vi "Qrcode Scanner Array Split.vi"() -> ()   [LabVIEW 2019]
uses:
  <vilib>/userDefined/High Color/IMAQdx.ctl
  <vilib>/vision/driver/NI_Vision_Acquisition_Software.lvlib
  <vilib>/vision/NI_Vision_Development_Module.lvlib
panel:
  out "Array":string[](array[string])
  in  "Session In":T1
  out "Found?":bool
  out "Image":T2(plugin-control)
  out "Data":string
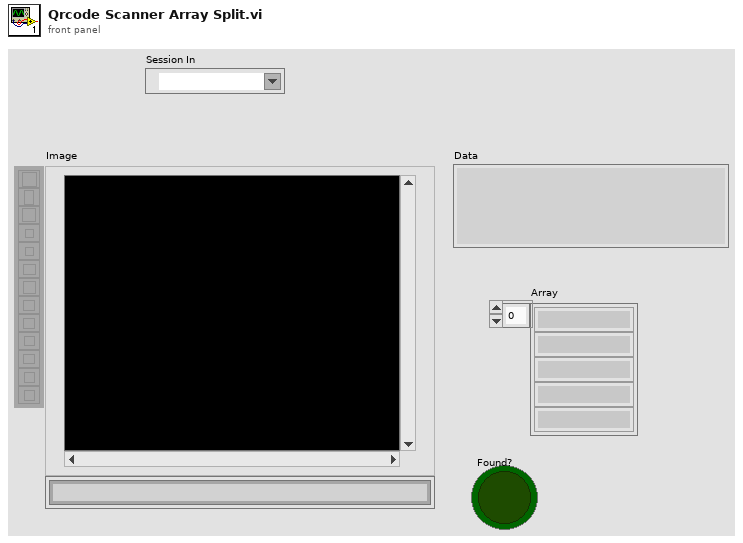
[diagram p1: front panel]
types:
  T1 = typedef "IMAQdx.ctl" = refnum<k21>
  T2 = typedef "IMAQ Image.ctl" = refnum<image>
  T3 = typedef "Image Type" = u32
  T4 = typedef "QR Code Report.ctl" = cluster{"Found?":bool, "Data":string, "Bounding Box":cluster{"x":sgl, "y":sgl}[], "Errors Corrected":u32, "Dimensions (Rows/Cols)":u32, "Version":u32, "QR Model":T5, "Stream Mode":T6, "Barcode Polarity":T7, "Mirrored?":bool, "Append Stream Position":u32, "Size of Append Stream":u32, "First EAN-128 ID":i32, "First Alternate Language ID":i32, "Append Stream ID":u32, "Minimum Edge Strength":u32, "Demodulation Mode":T8, "Cell Sample Size":T9, "Cell Filter Mode":T10}
  T5 = typedef "QR Code Model Type.ctl" = i32
  T6 = typedef "QR Code Stream Mode Type.ctl" = i32
  T7 = typedef "Data Matrix Polarity.ctl" = i32
  T8 = typedef "Demodulation Mode.ctl" = i32
  T9 = typedef "Cell Sample Size.ctl" = i32
  T10 = typedef "Cell Filter Mode.ctl" = i32
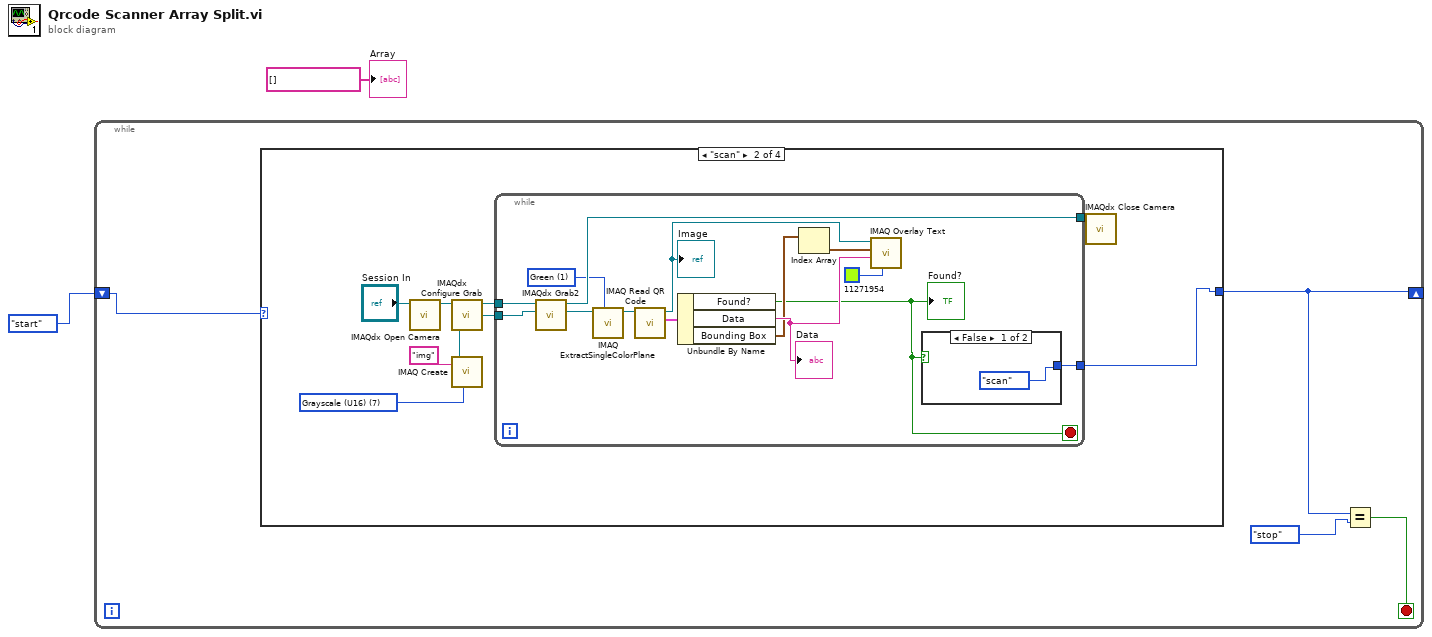
[diagram p0: block diagram]
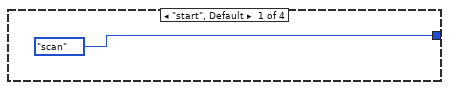
[diagram p2: hidden frame]
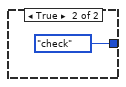
[diagram p3: hidden frame]
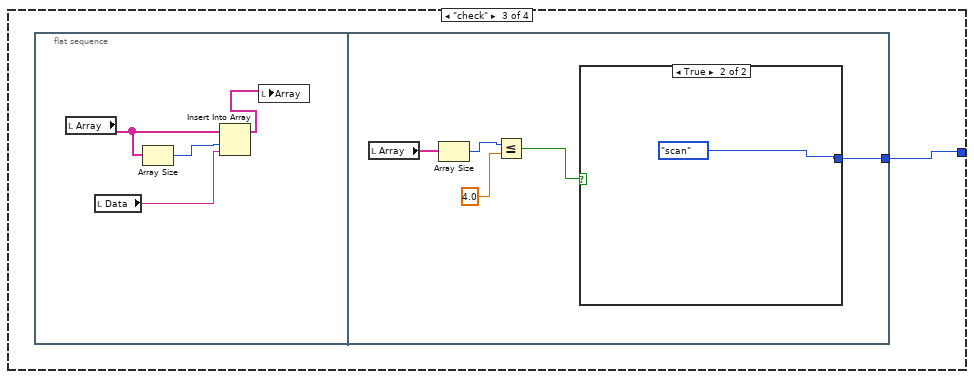
[diagram p4: hidden frame]
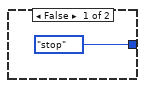
[diagram p5: hidden frame]
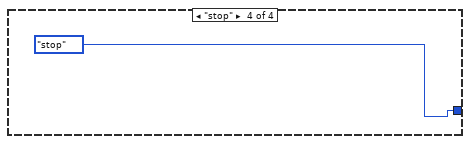
[diagram p6: hidden frame]
diagram:
  n1 = while {
    shift-right: [w3] -> _
    shift-left: enum16{"start", "scan", "check", "stop"}."start" -> [w6]
    stop <- w4 stop-if-true
    n2 = case shown="\"scan\"" w6 {
      tunnel: [enum16{"start", "scan", "check", "stop"}."scan" w8 w32 enum16{"start", "scan", "check", "stop"}."stop"] -> w3
      frame "start", Default {
      }
      frame "scan" {
        w10 = T3 7 items=["Grayscale (U8)", "Grayscale (I16)", "Grayscale (SGL)", "Complex (CSG)", "RGB (U32)", "HSL (U32)", "RGB (U64)", "Grayscale (U16)"] ("Image Type")
        n3 = call <vilib>:"IMAQdx Open Camera.vi"("Session In"="Session In") -> ("Session Out"=w14:T1)  [unwired: 9 in, 1 out]
        n4 = call <vilib>:"IMAQdx Configure Grab.vi"("Session In"=w14) -> ("Session Out"=w12:T1)  [unwired: 9 in, 1 out]
        n5 = call "IMAQ Create"("Image Name"="img", "Image Type"=w10) -> ("New Image"=w9:T2)  [unwired: 3 in, 1 out]
        n6 = while {
          tunnel: [w29] -> w13
          tunnel: w12 -> [w28]
          tunnel: w9 -> [w27]
          tunnel: [w16] -> w8
          stop <- w17 stop-if-true
          w24 = 1 items=["Red", "Green", "Blue", "Hue", "Saturation", "Luminance", "Value", "Intensity"] ("Color Plane")
          n7 = call <vilib>:"IMAQdx Grab2.vi"("Image In"=w27, "Session In"=w28) -> ("Image Out"=w26:T2, "Session Out"=w29:T1)  [unwired: 6 in, 2 out]
          n8 = call "IMAQ ExtractSingleColorPlane"("Color Plane"=w24, "Image Src"=w26) -> ("Image Dst Out"=w25:T2)  [unwired: 8 in, 1 out]
          n9 = call "IMAQ Read QR Code"("Image"=w25) -> ("QR Code Report"=w23:T4, "Image (duplicate)"=w18:T2)  [unwired: 7 in, 2 out]
          "Image" <- w18
          n10 = Unbundle By Name(w23) -> ("Found?"=w17:bool, "Data"=w21:string, "Bounding Box"=w19:cluster{"x":sgl, "y":sgl}[])
          "Found?" <- w17
          "Data" <- w21
          n11 = Index Array(array=w19) -> (element=w22:cluster{"x":sgl, "y":sgl})  [unwired: 1 in]
          n12 = call "IMAQ Overlay Text"("Text Color (black)"=u32 11271954, "String"=w21, "Origin"=w22, "Image"=w18) -> ()  [unwired: 6 in, 2 out]
          n13 = case shown="False" w17 {
            tunnel: [enum16{"start", "scan", "check", "stop"}."scan" enum16{"start", "scan", "check", "stop"}."check"] -> w16
            frame False {
            }
            frame True {
            }
          }
        }
        n14 = call <vilib>:"IMAQdx Close Camera.vi"("Session In"=w13) -> ()  [unwired: 10 in, 1 out]
      }
      frame "check" {
        n15 = flat-sequence {
          tunnel: [w38] -> w32
          frame #0 {
            n16 = local read "Array"() -> (w36:string[])
            n17 = local read "Data"() -> (w34:string)
            n18 = Array Size(array=w36) -> (size(s)=w35:i32)
            n19 = Insert Into Array(array=w36, index=w35, new element=w34) -> (w33:string[])
            n20 = local write "Array"(w33) -> ()
          }
          frame #1 {
            n21 = local read "Array"() -> (w40:string[])
            n22 = Array Size(array=w40) -> (size(s)=w39:i32)
            n23 = Less Or Equal?(x=w39, y=4.0) -> (x <= y?=w37:bool)
            n24 = case shown="True" w37 {
              tunnel: [enum16{"start", "scan", "check", "stop"}."stop" enum16{"start", "scan", "check", "stop"}."scan"] -> w38
              frame False {
              }
              frame True {
              }
            }
          }
        }
      }
      frame "stop" {
      }
    }
    n25 = Equal?(x=w3, y=enum16{"start", "scan", "check", "stop"}."stop") -> (x = y?=w4:bool)
  }
  "Array" <- string[] [] ("Array")
